vi "通讯调试.vi"() -> ()   [LabVIEW 2016]
uses:
  <vilib>/Plasmionique/MB Master/MB_Master/MB_Master.lvclass
  <vilib>/Plasmionique/MB Master/MB_Master_Serial/MB_Master_Serial.lvclass
  C:/Program Files (x86)/National Instruments/LabVIEW 2016/vi.lib/Plasmionique/MB Master/MB_Master/MB_Master.lvclass
  <vilib>/Plasmionique/MB Master/MB_Master_TCP/MB_Master_TCP.lvclass
  ESTD1200.lvlib
  <vilib>/Plasmionique/MB Master/MB Master.lvlib
panel:
  out "交换的字节":u16[](array[numeric]) format="%.0x"
  out "error out 2":errorcluster
  in  "VISA resource name":refnum<visa-resource-name>="COM3" caption="VISA资源名称"
  in  "写系统设置区":bool
  in  "启用模块":bool
  in  "系统复位":bool
  in  "软重启":bool
  in  "开门":bool
  in  "取样":bool
  in  "停止采样":bool
  in  "启动采样":bool
  in  "读取传感器实时浓度":bool
  in  "读取状态告警区":bool
  in  "读取系统设置区":bool
  in  "读取采样模式区":bool
  in  "读取采样状态区":bool
  out "传感器实时浓度":T1
  out "状态告警区":T2 {"告警代码" items=["无告警", "通讯异常(采样器与工控机通讯)", "滑台电机异常(过温/过流)", "蠕动泵异常(过温/过流)", "转盘电机异常(过温/过流)", "编码器异常", "转盘原点传感器异常", "滑台原点传感器异常", "冰箱温度异常", "冰箱通讯异常", "门禁锁异常", "串口屏通讯异常", "SD卡异常告警", "Flash异常告警(W25Q32)", "留样失败", "瓶满告警", "复位异常"]; "采样模式" items=["定时采样", "外控采样", "时间等比", "流量等比", "液位等比"]; "当前进程" items=["待机", "电机复位", "采样瓶转到采样区", "采样瓶排空", "采样泵管润洗", "采样瓶再排空", "采样", "采样泵反转排空管路", "取样瓶转到取样区"]}
  in  "系统设置区":T3
  out "采样模式区":T4 {"采样模式" items=["定时采样", "外控采样", "时间等比", "流量等比", "液位等比"]}
  out "采样状态区":T5 {"当前进程" items=["待机", "电机复位", "采样瓶转到采样区", "采样瓶排空", "采样泵管润洗", "采样瓶再排空", "采样", "采样泵反转排空管路", "取样瓶转到取样区"]; "采样模式" items=["定时采样", "外控采样", "时间等比", "流量等比", "液位等比"]; "采样器状态" items=["空闲", "忙碌"]}
  out "布尔":bool
  out "MB session in":refnum<class "MB_Master.lvclass">
  in  "Error in":errorcluster caption="Error in (no error)"
  out "error out":errorcluster
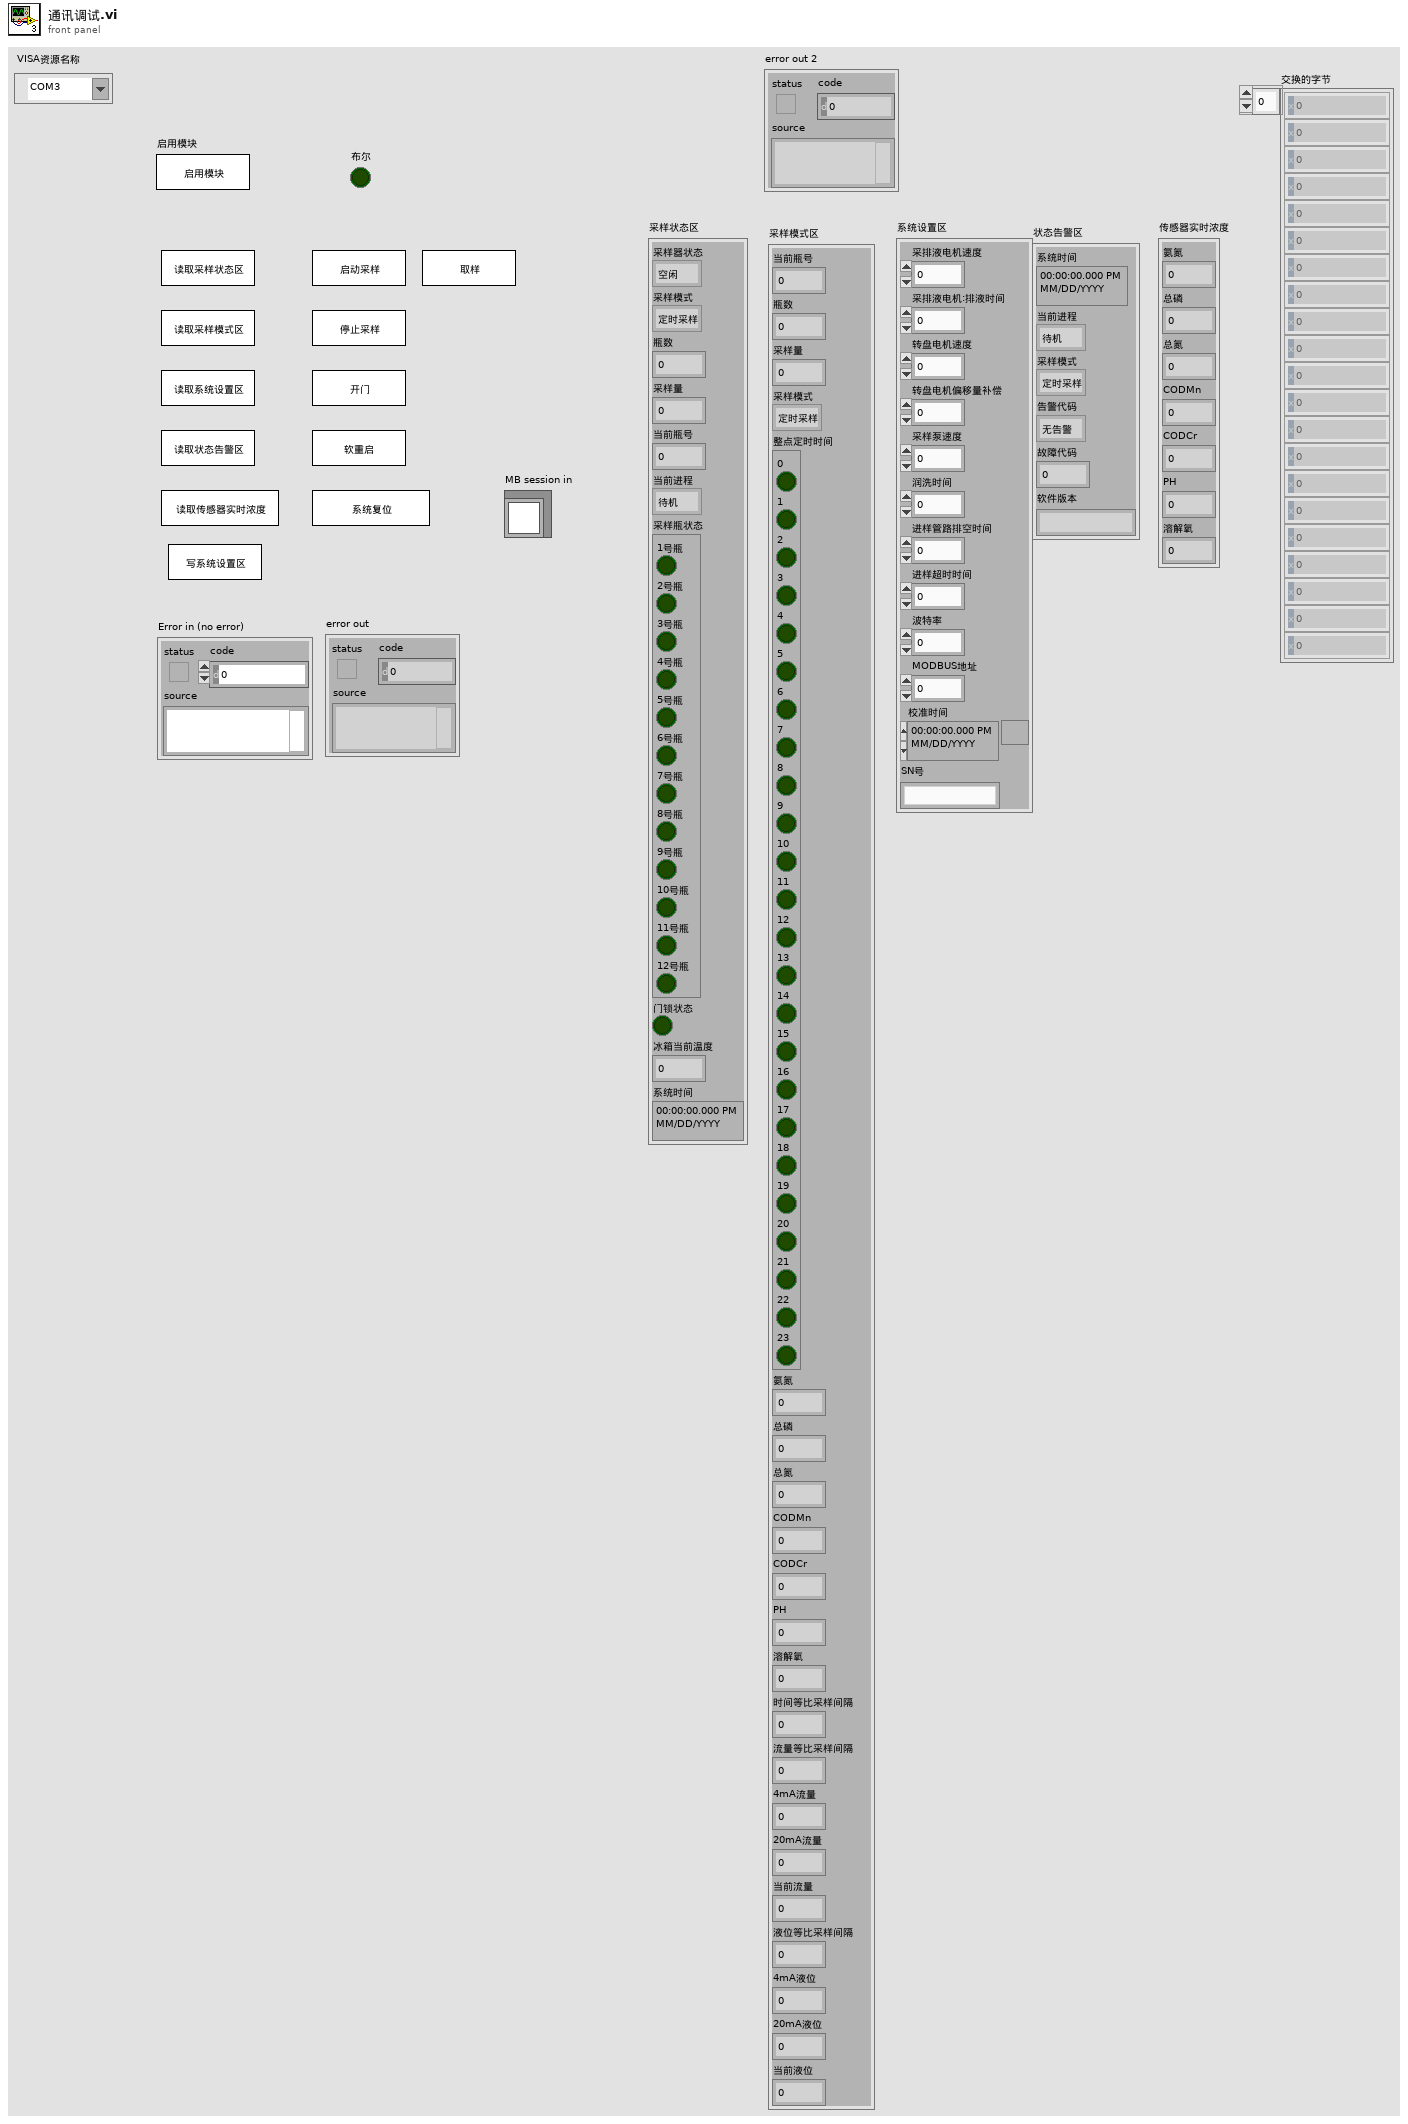
[diagram p1: front panel]
types:
  T1 = cluster{"氨氮":sgl, "总磷":sgl, "总氮":sgl, "CODMn":sgl, "CODCr":sgl, "PH":sgl, "溶解氧":sgl}
  T2 = cluster{"系统时间":timestamp, "当前进程":u16, "采样模式":u16, "告警代码":u16, "故障代码":u16, "软件版本":string}
  T3 = cluster{"采排液电机速度":u16, "采排液电机:排液时间":u16, "转盘电机速度":u16, "转盘电机偏移量补偿":u16, "采样泵速度":u16, "润洗时间":u16, "进样管路排空时间":u16, "进样超时时间":u16, "波特率":u16, "MODBUS地址":u16, "校准时间":timestamp, "SN号":string}
  T4 = cluster{"当前瓶号":u16, "瓶数":u16, "采样量":u16, "采样模式":u16, "整点定时时间":cluster{"0":bool, "1":bool, "2":bool, "3":bool, "4":bool, "5":bool, "6":bool, "7":bool, "8":bool, "9":bool, "10":bool, "11":bool, "12":bool, "13":bool, "14":bool, "15":bool, "16":bool, "17":bool, "18":bool, "19":bool, "20":bool, "21":bool, "22":bool, "23":bool}, "氨氮":sgl, "总磷":sgl, "总氮":sgl, "CODMn":sgl, "CODCr":sgl, "PH":sgl, "溶解氧":sgl, "时间等比采样间隔":u16, "流量等比采样间隔":sgl, "4mA流量":sgl, "20mA流量":sgl, "当前流量":sgl, "液位等比采样间隔":sgl, "4mA液位":sgl, "20mA液位":sgl, "当前液位":sgl}
  T5 = cluster{"采样器状态":u16, "采样模式":u16, "瓶数":u16, "采样量":u16, "当前瓶号":u16, "当前进程":u16, "采样瓶状态":cluster{"1号瓶":bool, "2号瓶":bool, "3号瓶":bool, "4号瓶":bool, "5号瓶":bool, "6号瓶":bool, "7号瓶":bool, "8号瓶":bool, "9号瓶":bool, "10号瓶":bool, "11号瓶":bool, "12号瓶":bool}, "门锁状态":bool, "冰箱当前温度":sgl, "系统时间":timestamp}
  T6 = typedef "队列data.ctl" = cluster{"命令":string, "data":cluster{"站号":u16, "控制命令":u16[]}}
  T7 = cluster{"命令":string, "data":cluster{"站号":u16, "控制命令":u16[]}}
  T8 = cluster{"baud rate (bps)":u32, "stop bits":u16, "parity":u16, "flow control":u16, "timeout":u32, "retries":i32}
  T9 = cluster{"[0]":bool, "[1]":bool, "[2]":bool, "[3]":bool, "[4]":bool, "[5]":bool, "[6]":bool, "[7]":bool, "[8]":bool, "[9]":bool, "[10]":bool, "[11]":bool}
  T10 = cluster{u16, u16, u16, u16, u16, u16, cluster{"[0]":bool, "[1]":bool, "[2]":bool, "[3]":bool, "[4]":bool, "[5]":bool, "[6]":bool, "[7]":bool, "[8]":bool, "[9]":bool, "[10]":bool, "[11]":bool}, bool, dbl, "time stamp":timestamp}
  T11 = cluster{"[0]":bool, "[1]":bool, "[2]":bool, "[3]":bool, "[4]":bool, "[5]":bool, "[6]":bool, "[7]":bool, "[8]":bool, "[9]":bool, "[10]":bool, "[11]":bool, "[12]":bool, "[13]":bool, "[14]":bool, "[15]":bool, "[16]":bool, "[17]":bool, "[18]":bool, "[19]":bool, "[20]":bool, "[21]":bool, "[22]":bool, "[23]":bool}
  T12 = cluster{u16, u16, u16, u16, cluster{"[0]":bool, "[1]":bool, "[2]":bool, "[3]":bool, "[4]":bool, "[5]":bool, "[6]":bool, "[7]":bool, "[8]":bool, "[9]":bool, "[10]":bool, "[11]":bool, "[12]":bool, "[13]":bool, "[14]":bool, "[15]":bool, "[16]":bool, "[17]":bool, "[18]":bool, "[19]":bool, "[20]":bool, "[21]":bool, "[22]":bool, "[23]":bool}, sgl, sgl, sgl, sgl, sgl, sgl, sgl, u16, sgl, sgl, sgl, sgl, sgl, sgl, sgl, sgl}
  T13 = cluster{u16, u16, u16, u16, u16, u16, u16, u16, u16, u16, "time stamp":timestamp, string}
  T14 = cluster{"time stamp":timestamp, u16, u16, u16, u16, string}
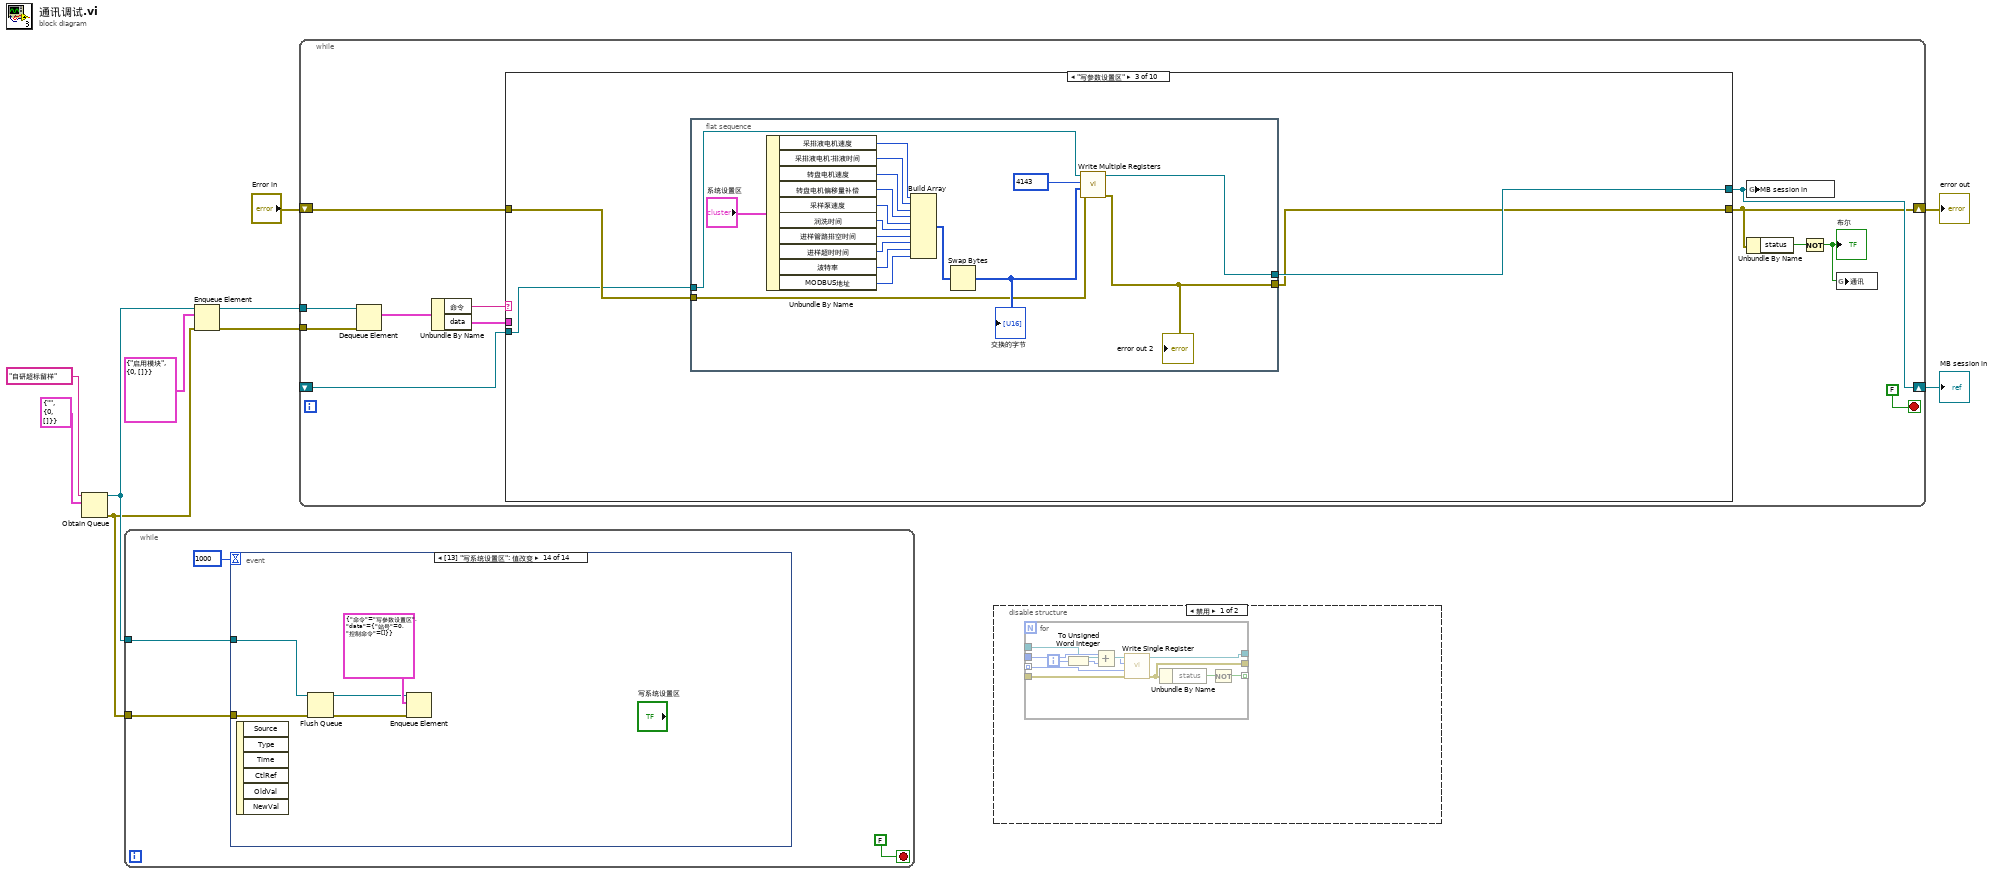
[diagram p0: block diagram]
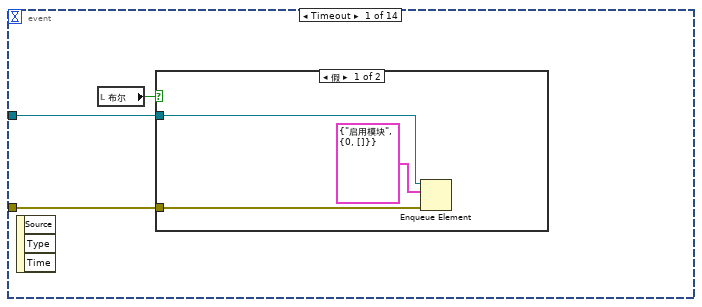
[diagram p3: hidden frame]
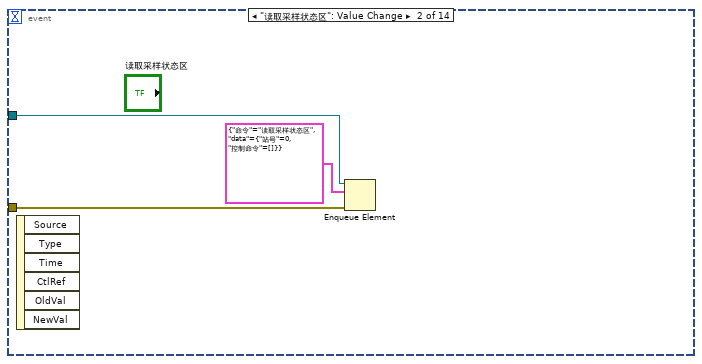
[diagram p5: hidden frame]
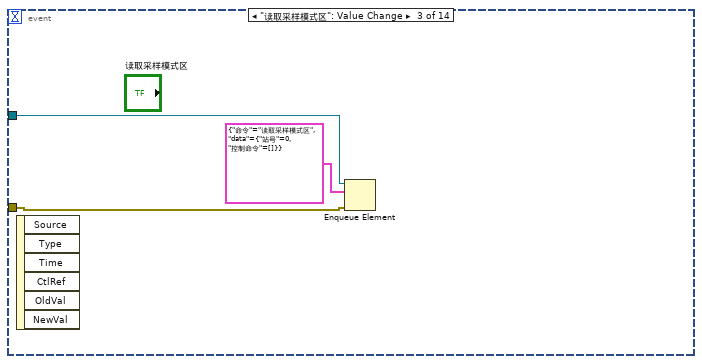
[diagram p6: hidden frame]
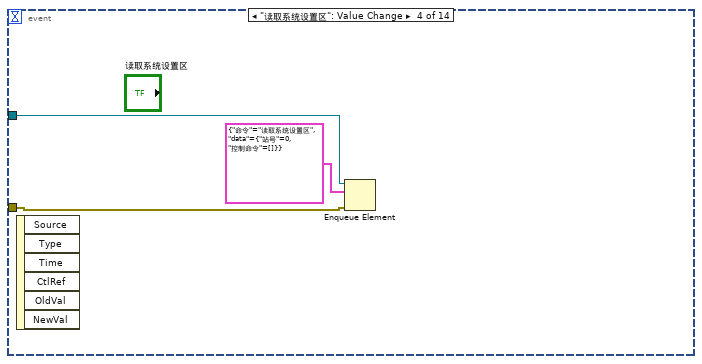
[diagram p7: hidden frame]
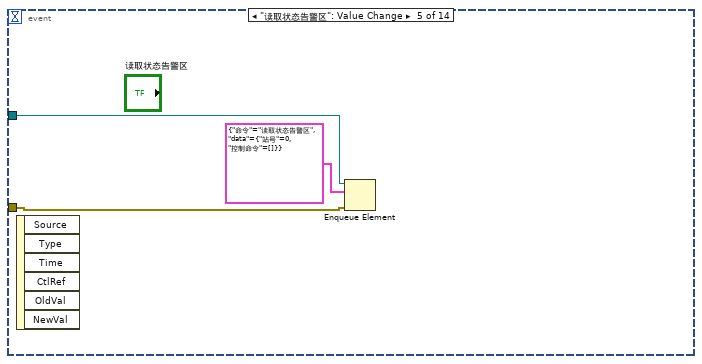
[diagram p8: hidden frame]
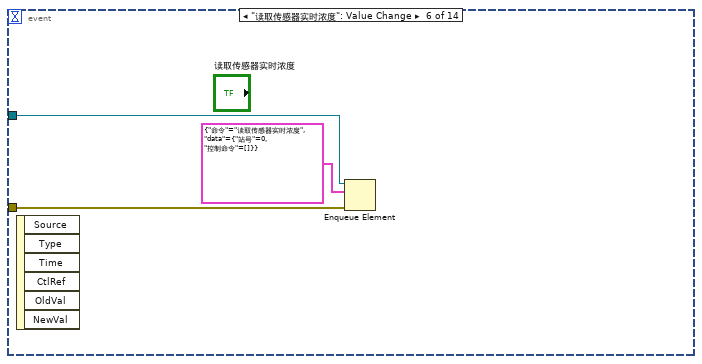
[diagram p9: hidden frame]
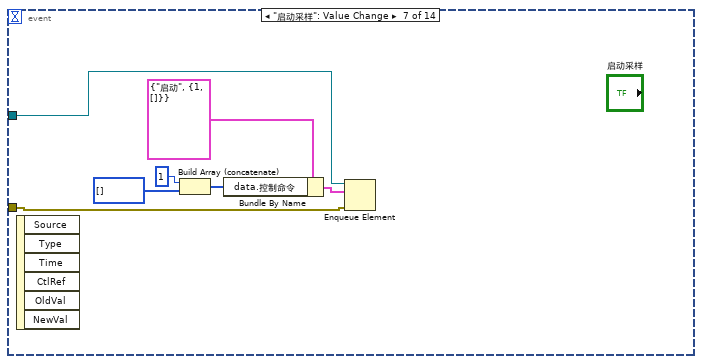
[diagram p10: hidden frame]
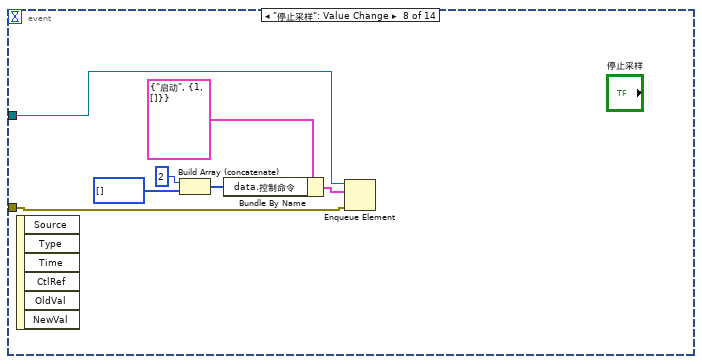
[diagram p11: hidden frame]
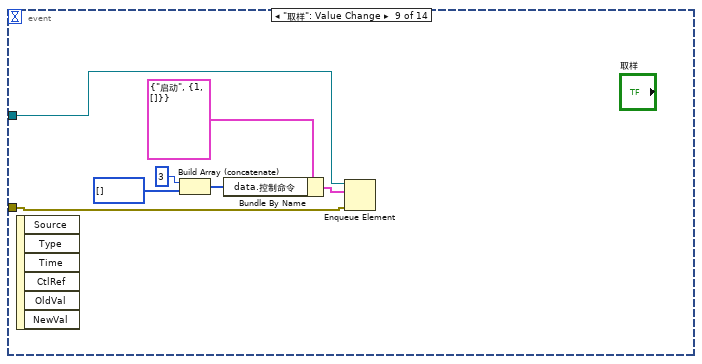
[diagram p12: hidden frame]
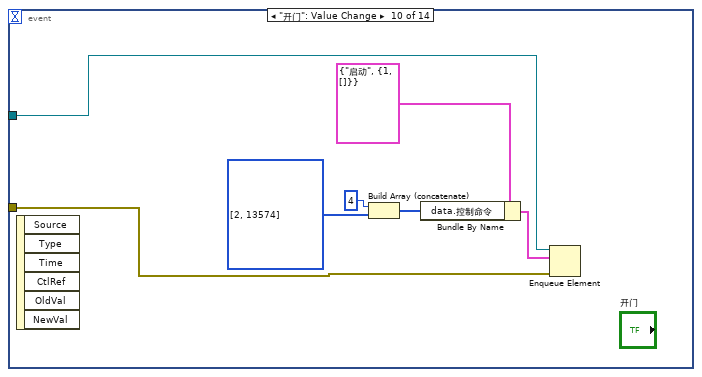
[diagram p13: hidden frame]
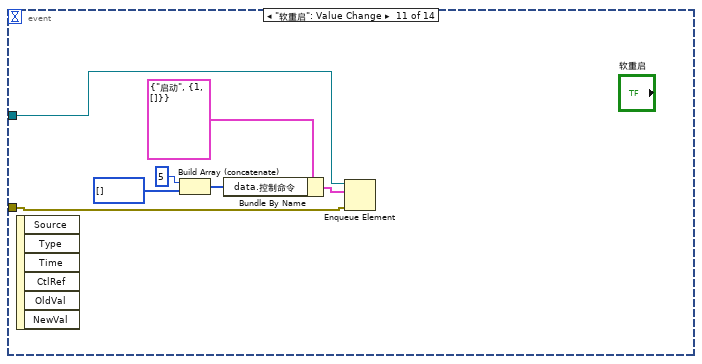
[diagram p14: hidden frame]
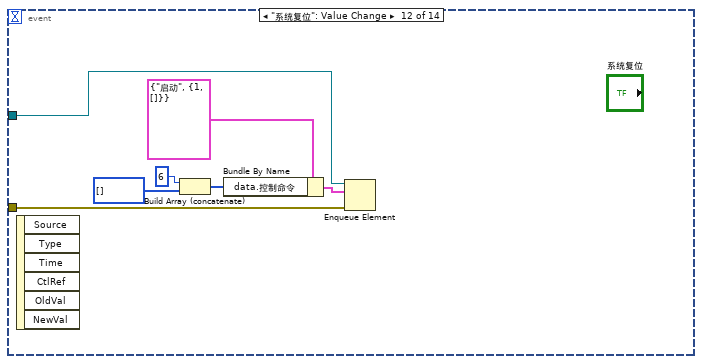
[diagram p15: hidden frame]
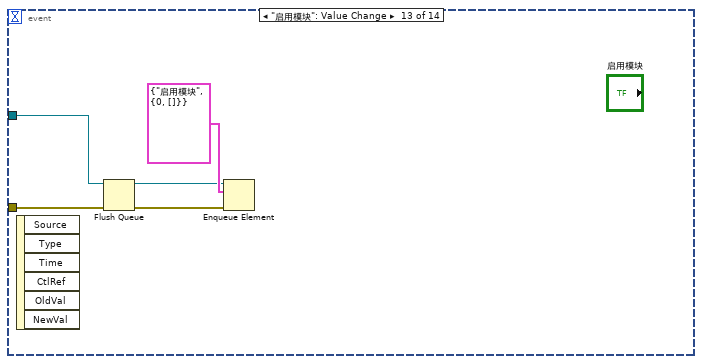
[diagram p16: hidden frame]
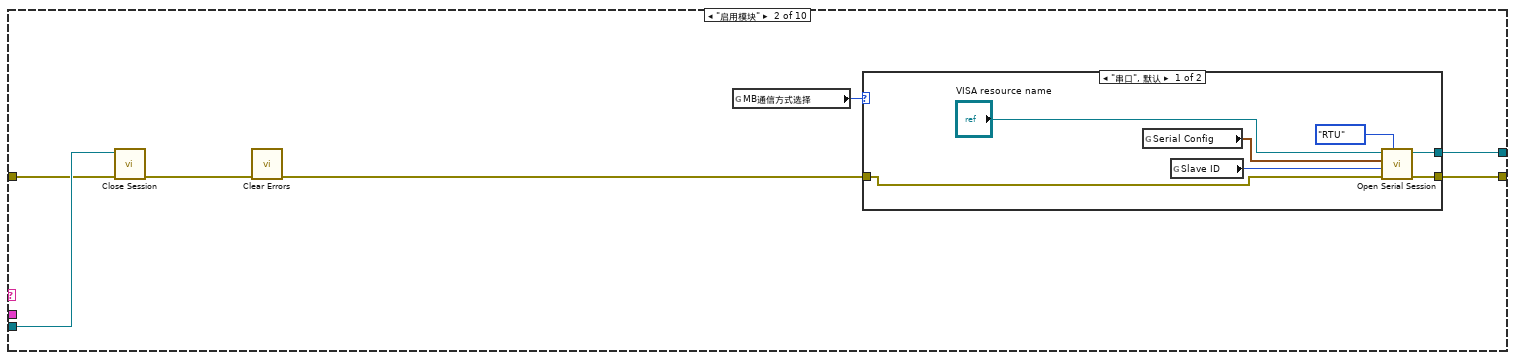
[diagram p18: hidden frame]
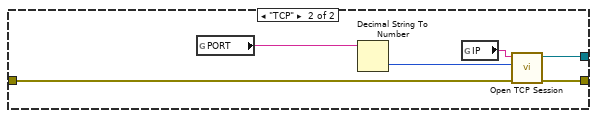
[diagram p19: hidden frame]
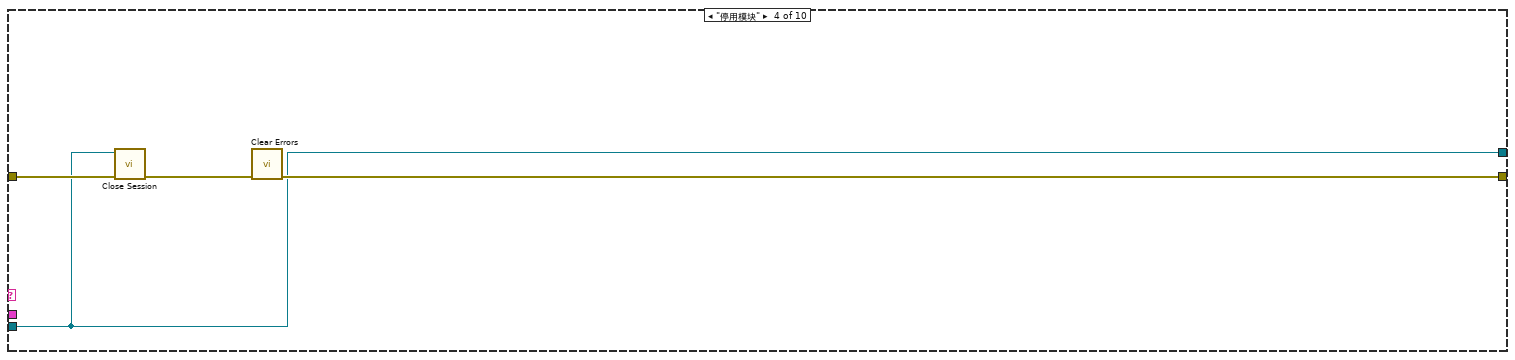
[diagram p20: hidden frame]
diagram:
  n1 = Obtain Queue(name (unnamed)="自研超标留样" ("名称（未命名）"), element data type=T6 {"命令"="", "data"={"站号"=0, "控制命令"=[]}}) -> (queue out=w5:refnum<queue>, error out=w4:errorcluster)  [unwired: 3 in, 1 out]
  n2 = while {
    tunnel: w5 -> [w13]
    tunnel: w4 -> [w12]
    stop <- FALSE stop-if-true
    n3 = event shown="[13] \"写系统设置区\": 值改变" {
      selector: _ -> [_ _ _ _ _ _ _ _ _ _ _ _ _ _]
      dyn-events: _ -> [_ _ _ _ _ _ _ _ _ _ _ _ _ _]
      timeout: 1000 -> [_ _ _ _ _ _ _ _ _ _ _ _ _ _]
      tunnel: w13 -> [w16 w23 w25 w28 w31 w34 w42 w45 w52 w59 w66 w73 w81 w86]
      tunnel: w12 -> [w15 w22 w24 w27 w30 w33 w41 w44 w51 w58 w65 w72 w79 w84]
      event Timeout {
        n4 = event-data() -> ()  [unwired: 1 in, 3 out]
        n5 = local read "布尔"() -> (w17:bool)
        n6 = case shown="假" w17 {
          tunnel: w16 -> [w20 _]
          tunnel: w15 -> [w19 _]
          frame False {
            n7 = Enqueue Element(queue=w20, element=T7 {"命令"="启用模块", "data"={"站号"=0, "控制命令"=[]}} ("元素"), error in (no error)=w19) -> ()  [unwired: 1 in, 3 out]
          }
          frame True {
          }
        }
      }
      event "读取采样状态区": Value Change {
        n8 = event-data() -> ()  [unwired: 1 in, 6 out]
        n9 = Enqueue Element(queue=w23, element=T7 {"命令"="读取采样状态区", "data"={"站号"=0, "控制命令"=[]}} ("元素"), error in (no error)=w22) -> ()  [unwired: 1 in, 3 out]
      }
      event "读取采样模式区": Value Change {
        n10 = event-data() -> ()  [unwired: 1 in, 6 out]
        n11 = Enqueue Element(queue=w25, element=T7 {"命令"="读取采样模式区", "data"={"站号"=0, "控制命令"=[]}} ("元素"), error in (no error)=w24) -> ()  [unwired: 1 in, 3 out]
      }
      event "读取系统设置区": Value Change {
        n12 = event-data() -> ()  [unwired: 1 in, 6 out]
        n13 = Enqueue Element(queue=w28, element=T7 {"命令"="读取系统设置区", "data"={"站号"=0, "控制命令"=[]}} ("元素"), error in (no error)=w27) -> ()  [unwired: 1 in, 3 out]
      }
      event "读取状态告警区": Value Change {
        n14 = event-data() -> ()  [unwired: 1 in, 6 out]
        n15 = Enqueue Element(queue=w31, element=T7 {"命令"="读取状态告警区", "data"={"站号"=0, "控制命令"=[]}} ("元素"), error in (no error)=w30) -> ()  [unwired: 1 in, 3 out]
      }
      event "读取传感器实时浓度": Value Change {
        n16 = event-data() -> ()  [unwired: 1 in, 6 out]
        n17 = Enqueue Element(queue=w34, element=T7 {"命令"="读取传感器实时浓度", "data"={"站号"=0, "控制命令"=[]}} ("元素"), error in (no error)=w33) -> ()  [unwired: 1 in, 3 out]
      }
      event "启动采样": Value Change {
        n18 = event-data() -> ()  [unwired: 1 in, 6 out]
        n19 = Build Array (concatenate)(u16 1 ("数值"), u16[] [] ("控制命令")) -> (w38:u16[])
        n20 = Bundle By Name(cluster=T7 {"命令"="启动", "data"={"站号"=1, "控制命令"=[]}} ("元素"), "data.控制命令"=w38) -> (w37:T7)
        n21 = Enqueue Element(queue=w42, element=w37, error in (no error)=w41) -> ()  [unwired: 1 in, 3 out]
      }
      event "停止采样": Value Change {
        n22 = event-data() -> ()  [unwired: 1 in, 6 out]
        n23 = Build Array (concatenate)(u16 2 ("数值"), u16[] [] ("控制命令")) -> (w47:u16[])
        n24 = Bundle By Name(cluster=T7 {"命令"="启动", "data"={"站号"=1, "控制命令"=[]}} ("元素"), "data.控制命令"=w47) -> (w46:T7)
        n25 = Enqueue Element(queue=w45, element=w46, error in (no error)=w44) -> ()  [unwired: 1 in, 3 out]
      }
      event "取样": Value Change {
        n26 = event-data() -> ()  [unwired: 1 in, 6 out]
        n27 = Build Array (concatenate)(u16 3 ("数值"), u16[] [] ("控制命令")) -> (w54:u16[])
        n28 = Bundle By Name(cluster=T7 {"命令"="启动", "data"={"站号"=1, "控制命令"=[]}} ("元素"), "data.控制命令"=w54) -> (w53:T7)
        n29 = Enqueue Element(queue=w52, element=w53, error in (no error)=w51) -> ()  [unwired: 1 in, 3 out]
      }
      event "开门": Value Change {
        n30 = event-data() -> ()  [unwired: 1 in, 6 out]
        n31 = Build Array (concatenate)(u16 4 ("数值"), u16[] [2, 13574] ("控制命令")) -> (w61:u16[])
        n32 = Bundle By Name(cluster=T7 {"命令"="启动", "data"={"站号"=1, "控制命令"=[]}} ("元素"), "data.控制命令"=w61) -> (w60:T7)
        n33 = Enqueue Element(queue=w59, element=w60, error in (no error)=w58) -> ()  [unwired: 1 in, 3 out]
      }
      event "软重启": Value Change {
        n34 = event-data() -> ()  [unwired: 1 in, 6 out]
        n35 = Build Array (concatenate)(u16 5 ("数值"), u16[] [] ("控制命令")) -> (w68:u16[])
        n36 = Bundle By Name(cluster=T7 {"命令"="启动", "data"={"站号"=1, "控制命令"=[]}} ("元素"), "data.控制命令"=w68) -> (w67:T7)
        n37 = Enqueue Element(queue=w66, element=w67, error in (no error)=w65) -> ()  [unwired: 1 in, 3 out]
      }
      event "系统复位": Value Change {
        n38 = event-data() -> ()  [unwired: 1 in, 6 out]
        n39 = Build Array (concatenate)(u16 6 ("数值"), u16[] [] ("控制命令")) -> (w75:u16[])
        n40 = Bundle By Name(cluster=T7 {"命令"="启动", "data"={"站号"=1, "控制命令"=[]}} ("元素"), "data.控制命令"=w75) -> (w74:T7)
        n41 = Enqueue Element(queue=w73, element=w74, error in (no error)=w72) -> ()  [unwired: 1 in, 3 out]
      }
      event "启用模块": Value Change {
        n42 = event-data() -> ()  [unwired: 1 in, 6 out]
        n43 = Flush Queue(queue=w81, error in (no error)=w79) -> (queue out=w80:refnum<queue>, error out=w78:errorcluster)  [unwired: 1 out]
        n44 = Enqueue Element(queue=w80, element=T7 {"命令"="启用模块", "data"={"站号"=0, "控制命令"=[]}} ("元素"), error in (no error)=w78) -> ()  [unwired: 1 in, 3 out]
      }
      event "写系统设置区": Value Change {
        n45 = event-data() -> ()  [unwired: 1 in, 6 out]
        n46 = Flush Queue(queue=w86, error in (no error)=w84) -> (queue out=w85:refnum<queue>, error out=w83:errorcluster)  [unwired: 1 out]
        n47 = Enqueue Element(queue=w85, element=T7 {"命令"="写参数设置区", "data"={"站号"=0, "控制命令"=[]}} ("元素"), error in (no error)=w83) -> ()  [unwired: 1 in, 3 out]
      }
    }
  }
  n48 = Enqueue Element(queue=w5, element=T7 {"命令"="启用模块", "data"={"站号"=0, "控制命令"=[]}} ("元素"), error in (no error)=w4) -> (queue out=w3:refnum<queue>, error out=w2:errorcluster)  [unwired: 1 in, 1 out]
  n49 = while {
    tunnel: w3 -> [w99]
    tunnel: w2 -> [w98]
    shift-right: [w94] -> w7
    shift-left: _ -> [w97]
    shift-right: [w89] -> w8
    shift-left: "Error in" -> [w96]
    stop <- FALSE stop-if-true
    n50 = Dequeue Element(queue=w99, error in (no error)=w98) -> (element=w93:T6)  [unwired: 1 in, 3 out]
    n51 = Unbundle By Name(w93) -> ("命令"=w92:string, "data"=w91:cluster{"站号":u16, "控制命令":u16[]})
    n52 = case shown="\"写参数设置区\"" w92 {
      tunnel: [w101 w105 w123 w144 w149 w189 w243 w260 w303 w341] -> w94
      tunnel: w97 -> [w101 w104 w124 w144 w152 w191 w247 w286 w328 w344]
      tunnel: [w100 w103 w122 w145 w148 w188 w242 w259 w302 w340] -> w89
      tunnel: w96 -> [w100 w102 w125 w146 w151 w190 w246 w285 w327 w343]
      tunnel: w91 -> [_ _ _ _ w158 _ _ _ _ _]
      frame "", Default {
      }
      frame "启用模块" {
        n53 = call-dynamic "Close Session.vi"("error in (no error)"=w102, "MB session in"=w104) -> ("error out"=w108:errorcluster)  [unwired: 9 in]
        n54 = call <vilib>:"Clear Errors.vi"("error in (no error)"=w108) -> ("error out"=w107:errorcluster)  [unwired: 5 in, 1 out]
        n55 = global read "串口参数断电保存全局变量.vi" "MB通信方式选择"() -> (w106:enum16{"串口", "TCP"})
        n56 = case shown="\"串口\", 默认" w106 {
          tunnel: [w114 w120] -> w103
          tunnel: [w110 w118] -> w105
          tunnel: w107 -> [w113 w119]
          frame "串口", Default {
            n57 = global read "串口参数断电保存全局变量.vi" "Serial Config"() -> (w111:T8)
            n58 = global read "串口参数断电保存全局变量.vi" "Slave ID"() -> (w112:u8)
            n59 = call <vilib>:"Open Serial Session.vi"("Mode (RTU)"=enum16{"RTU", "ASCII"}."RTU", "Error in"=w113, "Slave ID"=w112, "Serial Config"=w111, "VISA Resource"="VISA resource name") -> ("Error out"=w114:errorcluster, "MB_Serial session"=w110:refnum<class "MB_Master_Serial.lvclass">)  [unwired: 5 in]
          }
          frame "TCP" {
            n60 = global read "串口参数断电保存全局变量.vi" "PORT"() -> (w116:string)
            n61 = Decimal String To Number(string=w116) -> (number=w121:i32)  [unwired: 2 in, 1 out]
            n62 = global read "串口参数断电保存全局变量.vi" "IP"() -> (w117:string)
            n63 = call <vilib>:"Open TCP Session.vi"("error in (no error)"=w119, "Port (502)"=w121, "IP Address"=w117) -> ("error out"=w120:errorcluster, "MB_TCP session"=w118:refnum<class "MB_Master_TCP.lvclass">)  [unwired: 7 in]
          }
        }
      }
      frame "写参数设置区" {
        n64 = flat-sequence {
          tunnel: w125 -> [w126]
          tunnel: w124 -> [w127]
          tunnel: [w131] -> w123
          tunnel: [w130] -> w122
          frame #0 {
            n65 = Unbundle By Name("系统设置区") -> ("采排液电机速度"=w142:u16, "采排液电机:排液时间"=w141:u16, "转盘电机速度"=w140:u16, "转盘电机偏移量补偿"=w139:u16, "采样泵速度"=w138:u16, "润洗时间"=w137:u16, "进样管路排空时间"=w136:u16, "进样超时时间"=w135:u16, "波特率"=w134:u16, "MODBUS地址"=w133:u16)
            n66 = Build Array(w142, w141, w140, w139, w138, w137, w136, w135, w134, w133) -> (w132:u16[])
            n67 = Swap Bytes(anything=w132) -> (byte swapped=w128:u16[])
            "交换的字节" <- w128
            n68 = call <vilib>:"Write Multiple Registers.vi"("error in (no error)"=w126, "values"=w128, "starting address"=u16 4143, "MB session in"=w127) -> ("error out"=w130:errorcluster, "MB session out"=w131:refnum<class "MB_Master.lvclass">)  [unwired: 6 in]
            "error out 2" <- w130
          }
        }
      }
      frame "停用模块" {
        n69 = call-dynamic "Close Session.vi"("error in (no error)"=w146, "MB session in"=w144) -> ("error out"=w147:errorcluster)  [unwired: 9 in]
        n70 = call <vilib>:"Clear Errors.vi"("error in (no error)"=w147) -> ("error out"=w145:errorcluster)  [unwired: 5 in, 1 out]
      }
      frame "启动" {
        n71 = Unbundle By Name(w158) -> ("站号"=w153:u16, "控制命令"=w150:u16[])
        n72 = property class="MB_Master"(reference=w152, error in=w151, "Properties:Slave ID"=w153) -> (reference out=w155:refnum<class "MB_Master.lvclass">, error out=w154:errorcluster)
        n73 = Index Array(array=w150) -> (element=w157:u16)  [unwired: 1 in]
        n74 = Swap Bytes(anything=w157) -> ()  [unwired: 1 out]
        n75 = call <vilib>:"Write Multiple Registers.vi"("error in (no error)"=w154, "values"=w150, "starting address"=u16 80, "MB session in"=w155) -> ("error out"=w148:errorcluster, "MB session out"=w149:refnum<class "MB_Master.lvclass">)  [unwired: 6 in]
      }
      frame "读取采样状态区" {
        n76 = call <vilib>:"Read Holding Registers.vi"("error in (no error)"=w190, "quantity"=u16 20, "starting address"=u16 0, "MB session in"=w191) -> ("error out"=w188:errorcluster, "Registers"=w163:u16[], "MB session out"=w189:refnum<class "MB_Master.lvclass">)  [unwired: 5 in]
        n77 = call "HexToWord.vi"("Registers"=w163) -> ("数组"=w159:u16[])  [unwired: 10 in]
        n78 = Array Subset(array=w163, index=6 ("索引"), length=6 ("长度")) -> (w174:u16[])
        n79 = Array Subset(array=w163, index=14 ("索引"), length=3 ("长度")) -> (w167:u16[])
        n80 = for {
          tunnel: w174 -> [w199] mode=indexing
          shift-right: [w195] -> w176
          shift-left: u8[] [] -> [w196]
          n81 = Split Number(x=w199) -> (hi(x)=w198:u8, lo(x)=w197:u8)
          n82 = Build Array(w198, w197) -> (w194:u8[])
          n83 = Insert Into Array(array=w196, new element=w194) -> (w195:u8[])  [unwired: 1 in]
        }
        n84 = call "HexToDate.vi"("数组输入"=w167) -> ("数组输出"=w166:timestamp[])  [unwired: 10 in]
        n85 = Index Array(array=w166) -> (element=w165:timestamp)  [unwired: 1 in]
        n86 = for {
          tunnel: w176 -> [w193] mode=indexing
          tunnel: [w192] -> w175 mode=indexing
          n87 = Not Equal To 0?(x=w193) -> (x != 0?=w192:bool)
        }
        n88 = Index Array(array=w159, index #7=12 ("索引")) -> (element #1=w185:u16, element #2=w184:u16, element #3=w183:u16, element #4=w182:u16, element #5=w181:u16, element #6=w180:u16, element #7=w171:u16, element #8=w162:u16)  [unwired: 7 in]
        n89 = Divide(x=w162, y=u16 10) -> (x/y=w160:dbl)
        n90 = Not Equal To 0?(x=w171) -> (x != 0?=w170:bool)
        n91 = Array To Cluster(array=w175) -> (cluster=w173:T9)
        n92 = Bundle(w185, w184, w183, w182, w181, w180, w173, w170, w160, "time stamp"=w165) -> (w164:T10)  [unwired: 1 in]
        "采样状态区" <- w164
        n93 = global write "超标留样全局.vi" "采样状态区"(w164) -> ()
      }
      frame "读取采样模式区" {
        n94 = call <vilib>:"Read Holding Registers.vi"("error in (no error)"=w246, "quantity"=u16 46, "starting address"=u16 4096, "MB session in"=w247) -> ("error out"=w242:errorcluster, "Registers"=w201:u16[], "MB session out"=w243:refnum<class "MB_Master.lvclass">)  [unwired: 5 in]
        n95 = Array Subset(array=w201, index=4 ("索引"), length=12 ("长度")) -> (w232:u16[])
        n96 = Array Subset(array=w201, index=16 ("索引"), length=14 ("长度")) -> (w227:u16[])
        n97 = Array Subset(array=w201, index=31 ("索引"), length=16 ("长度")) -> (w214:u16[])
        n98 = call "HexToFloat.vi"("数组输入"=w227) -> ("数组输出"=w226:sgl[])  [unwired: 10 in]
        n99 = call "HexToFloat.vi"("数组输入"=w214) -> ("数组输出"=w211:sgl[])  [unwired: 10 in]
        n100 = for {
          tunnel: w232 -> [w257] mode=indexing
          shift-right: [w253] -> w236
          shift-left: u8[] [] -> [w254]
          n101 = Split Number(x=w257) -> (hi(x)=w256:u8, lo(x)=w255:u8)
          n102 = Build Array(w256, w255) -> (w252:u8[])
          n103 = Insert Into Array(array=w254, new element=w252) -> (w253:u8[])  [unwired: 1 in]
        }
        n104 = call "HexToWord.vi"("Registers"=w201) -> ("数组"=w200:u16[])  [unwired: 10 in]
        n105 = for {
          tunnel: w236 -> [w251] mode=indexing
          tunnel: [w250] -> w231 mode=indexing
          n106 = Not Equal To 0?(x=w251) -> (x != 0?=w250:bool)
        }
        n107 = Array Subset(array=w200, index=0 ("索引"), length=4 ("长度")) -> (w235:u16[])
        n108 = Array Subset(array=w200, index=30 ("索引"), length=1 ("长度")) -> (w216:u16[])
        n109 = Index Array(array=w216) -> (element=w215:u16)  [unwired: 1 in]
        n110 = Array To Cluster(array=w231) -> (cluster=w230:T11)
        n111 = Index Array(array=w235) -> (element #1=w241:u16, element #2=w240:u16, element #3=w239:u16, element #4=w238:u16)  [unwired: 4 in]
        n112 = Index Array(array=w226) -> (element #1=w225:sgl, element #2=w224:sgl, element #3=w223:sgl, element #4=w222:sgl, element #5=w221:sgl, element #6=w220:sgl, element #7=w219:sgl)  [unwired: 7 in]
        n113 = Index Array(array=w211) -> (element #1=w210:sgl, element #2=w209:sgl, element #3=w208:sgl, element #4=w207:sgl, element #5=w206:sgl, element #6=w205:sgl, element #7=w204:sgl, element #8=w203:sgl)  [unwired: 8 in]
        n114 = Bundle(w241, w240, w239, w238, w230, w225, w224, w223, w222, w221, w220, w219, w215, w210, w209, w208, w207, w206, w205, w204, w203) -> (w202:T12)  [unwired: 1 in]
        "采样模式区" <- w202
        n115 = global write "超标留样全局.vi" "采样模式区"(w202) -> ()
      }
      frame "读取系统设置区" {
        n116 = call <vilib>:"Read Holding Registers.vi"("error in (no error)"=w285, "quantity"=u16 18, "starting address"=u16 4143, "MB session in"=w286) -> ("error out"=w259:errorcluster, "Registers"=w264:u16[], "MB session out"=w260:refnum<class "MB_Master.lvclass">)  [unwired: 5 in]
        n117 = call "HexToWord.vi"("Registers"=w264) -> ("数组"=w284:u16[])  [unwired: 10 in]
        n118 = Array Subset(array=w264, index=10 ("索引"), length=3 ("长度")) -> (w271:u16[])
        n119 = Array Subset(array=w264, index=13 ("索引"), length=6 ("长度")) -> (w265:u16[])
        n120 = call "HexToDate.vi"("数组输入"=w271) -> ("数组输出"=w270:timestamp[])  [unwired: 10 in]
        n121 = for {
          tunnel: w265 -> [w298] mode=indexing
          shift-right: [w294] -> w263
          shift-left: u8[] [] -> [w295]
          n122 = Split Number(x=w298) -> (hi(x)=w297:u8, lo(x)=w296:u8)
          n123 = Build Array(w297, w296) -> (w293:u8[])
          n124 = Insert Into Array(array=w295, new element=w293) -> (w294:u8[])  [unwired: 1 in]
        }
        n125 = Index Array(array=w270) -> (element=w269:timestamp)  [unwired: 1 in]
        n126 = for {
          tunnel: w263 -> [w292] mode=indexing
          shift-right: [w289] -> w261
          shift-left: "" -> [w290]
          n127 = Number To Decimal String(number=w292) -> (decimal integer string=w291:string)  [unwired: 1 in]
          n128 = Concatenate Strings(w290, w291) -> (w289:string)
        }
        n129 = Index Array(array=w284) -> (element #1=w283:u16, element #2=w282:u16, element #3=w281:u16, element #4=w280:u16, element #5=w279:u16, element #6=w278:u16, element #7=w277:u16, element #8=w276:u16, element #9=w275:u16, element #10=w274:u16)  [unwired: 10 in]
        n130 = Bundle(w283, w282, w281, w280, w279, w278, w277, w276, w275, w274, "time stamp"=w269, w261) -> (w258:T13)  [unwired: 1 in]
        n131 = global write "超标留样全局.vi" "系统设置区"(w258) -> ()
        n132 = local write "系统设置区"(w258) -> ()
      }
      frame "读取状态告警区" {
        n133 = call <vilib>:"Read Holding Registers.vi"("error in (no error)"=w327, "quantity"=u16 14, "starting address"=u16 4224, "MB session in"=w328) -> ("error out"=w304:errorcluster, "Registers"=w312:u16[], "MB session out"=w305:refnum<class "MB_Master.lvclass">)  [unwired: 5 in]
        n134 = call "HexToWord.vi"("Registers"=w312) -> ("数组"=w319:u16[])  [unwired: 10 in]
        n135 = Array Subset(array=w312, index=0 ("索引"), length=3 ("长度")) -> (w324:u16[])
        n136 = Array Subset(array=w312, index=7 ("索引"), length=8 ("长度")) -> (w311:u16[])
        n137 = call "HexToDate.vi"("数组输入"=w324) -> ("数组输出"=w323:timestamp[])  [unwired: 10 in]
        n138 = call "HexToString.vi"("数组输入"=w311) -> ("数组输出"=w310:string[])  [unwired: 10 in]
        n139 = call <vilib>:"Read Holding Registers.vi"("error in (no error)"=w304, "quantity"=u16 1, "starting address"=u16 17, "MB session in"=w305) -> ("error out"=w302:errorcluster, "Registers"=w301:u16[], "MB session out"=w303:refnum<class "MB_Master.lvclass">)  [unwired: 5 in]
        n140 = call "HexToWord.vi"("Registers"=w301) -> ("数组"=w300:u16[])  [unwired: 10 in]
        n141 = Index Array(array=w323) -> (element=w322:timestamp)  [unwired: 1 in]
        n142 = Array Subset(array=w319, index=3 ("索引"), length=4 ("长度")) -> (w318:u16[])
        n143 = Index Array(array=w318) -> (element #1=w317:u16, element #2=w316:u16, element #4=w315:u16)  [unwired: 4 in, 1 out]
        n144 = Index Array(array=w310) -> (element=w309:string)  [unwired: 1 in]
        n145 = Index Array(array=w300) -> (element=w299:u16)  [unwired: 1 in]
        n146 = Bundle("time stamp"=w322, w317, w316, w299, w315, w309) -> (w308:T14)  [unwired: 1 in]
        "状态告警区" <- w308
        n147 = global write "超标留样全局.vi" "状态告警区"(w308) -> ()
      }
      frame "读取传感器实时浓度" {
        n148 = call <vilib>:"Read Holding Registers.vi"("error in (no error)"=w343, "quantity"=u16 14, "starting address"=u16 128, "MB session in"=w344) -> ("error out"=w340:errorcluster, "Registers"=w342:u16[], "MB session out"=w341:refnum<class "MB_Master.lvclass">)  [unwired: 5 in]
        n149 = call "HexToFloat.vi"("数组输入"=w342) -> ("数组输出"=w339:sgl[])  [unwired: 10 in]
        n150 = Index Array(array=w339) -> (element #1=w338:sgl, element #2=w337:sgl, element #3=w336:sgl, element #4=w335:sgl, element #5=w334:sgl, element #6=w333:sgl, element #7=w332:sgl)  [unwired: 7 in]
        n151 = Bundle(w338, w337, w336, w335, w334, w333, w332) -> (w331:cluster{sgl, sgl, sgl, sgl, sgl, sgl, sgl})  [unwired: 1 in]
        "传感器实时浓度" <- w331
        n152 = global write "超标留样全局.vi" "传感器实时浓度"(w331) -> ()
      }
    }
    n153 = global write "超标留样全局.vi" "MB session in"(w94) -> ()
    n154 = Unbundle By Name(w89) -> ("status"=w90:bool)
    n155 = Not(x=w90) -> (.not. x?=w88:bool)
    "布尔" <- w88
    n156 = global write "超标留样全局.vi" "通讯"(w88) -> ()
  }
  "error out" <- w8
  "MB session in" <- w7
  n157 = disable-structure shown="禁用" {
    frame Disabled {
      n158 = for {
        tunnel: _ -> [w357] mode=indexing
        tunnel: _ -> [w356]
        tunnel: _ -> [w355]
        tunnel: _ -> [w354]
        tunnel: [w353] -> _
        tunnel: [w351] -> _
        tunnel: [w350] -> _ mode=indexing
        i -> [w349]
        n159 = To Unsigned Word Integer(number=w349) -> (unsigned 16bit integer=w348:u16)
        n160 = Add(x=w356, y=w348) -> (x+y=w347:u16)
        n161 = call <vilib>:"Write Single Register.vi"("error in (no error)"=w355, "value"=w357, "address"=w347, "MB session in"=w354) -> ("error out"=w351:errorcluster, "MB session out"=w353:refnum<class "MB_Master.lvclass">)  [unwired: 6 in]
        n162 = Unbundle By Name(w351) -> ("status"=w352:bool)
        n163 = Not(x=w352) -> (.not. x?=w350:bool)
      }
    }
    frame Enabled {
    }
  }
